vi "DataTypesDetect.vi"(1 "input data":cluster{"name":string, "type desc":i16[]}[](array[cluster])) -> (0 "output data":cluster{"name":string, "type desc":i16[]}[](array[cluster]))   [LabVIEW 2010]
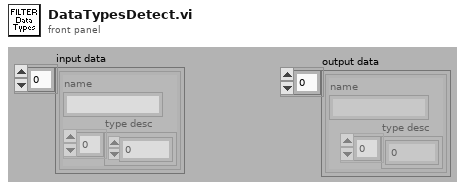
[diagram p1: front panel]
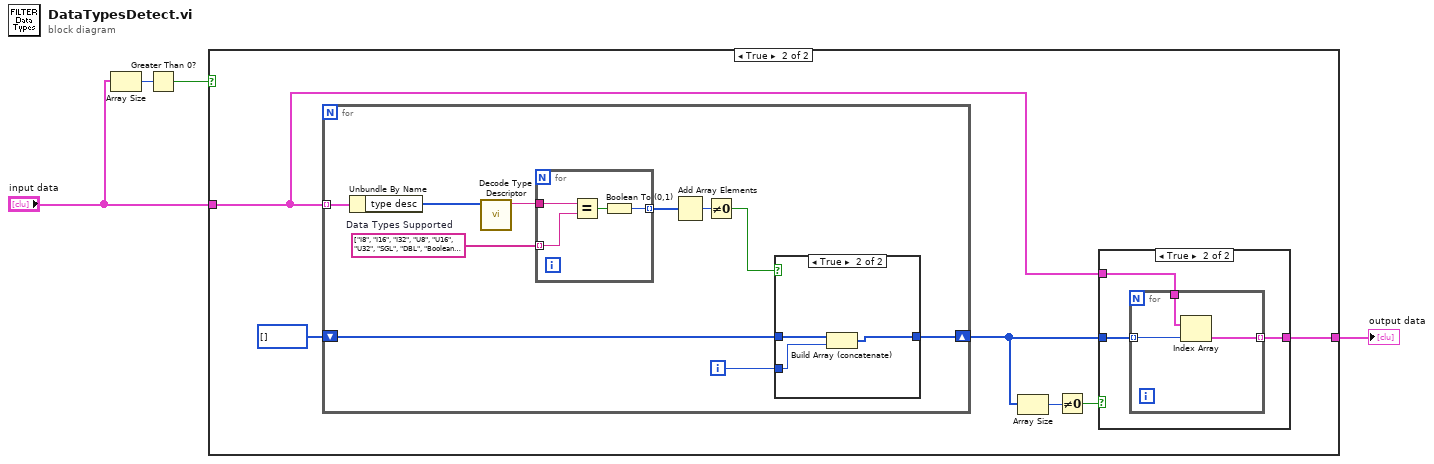
[diagram p0: block diagram]
diagram:
  n1 = Array Size(array="input data") -> (size(s)=w2:i32)
  n2 = Greater Than 0?(x=w2) -> (x > 0?=w3:bool)
  n3 = case shown="True" w3 {
    tunnel: [w5 w11] -> w4
    tunnel: "input data" -> [w5 w8]
    frame False {
    }
    frame True {
      n4 = for {
        tunnel: w8 -> [w27] mode=indexing
        shift-right: [w23] -> w9
        shift-left: i32[] [] -> [w24]
        i -> [w22]
        w21 = string[] ["I8", "I16", "I32", "U8", "U16", "U32", "SGL", "DBL", "Boolean", "String", "Array1D(I8)", "Array1D(I16)", "Array1D(I32)", "Array1D(U8)", "Array1D(U16)", "Array1D(U32)", "Array1D(SGL)", "Array1D(DBL)", "Array1D(Boolean)", "Array1D(String)", "Array2D(I8)", "Array2D(I16)", "Array2D(I32)", "Array2D(U8)", "Array2D(U16)", "Array2D(U32)", "Array2D(SGL)", "Array2D(DBL)", "Array2D(Boolean)", "Array2D(String)"]  # Data Types Supported
        n5 = Unbundle By Name(w27) -> ("type desc"=w20:i16[])
        n6 = call "Decode Type Descriptor.vi"("TypeDesc"=w20) -> ("Type String"=w19:string)  [unwired: 1 in, 5 out]
        n7 = for {
          tunnel: w21 -> [w35] mode=indexing
          tunnel: w19 -> [w36]
          tunnel: [w33] -> w28 mode=indexing
          n8 = Equal?(x=w36, y=w35) -> (x = y?=w34:bool)
          n9 = Boolean To (0,1)(Boolean=w34) -> (0, 1=w33:i16)
        }
        n10 = Add Array Elements(numeric array=w28) -> (sum=w26:i16)
        n11 = Not Equal To 0?(x=w26) -> (x != 0?=w25:bool)
        n12 = case shown="True" w25 {
          tunnel: w24 -> [w29 w32]
          tunnel: [w29 w30] -> w23
          tunnel: w22 -> [_ w31]
          frame False {
          }
          frame True {
            n13 = Build Array (concatenate)(w32, w31) -> (w30:i32[])
          }
        }
      }
      n14 = Array Size(array=w9) -> (size(s)=w6:i32)
      n15 = Not Equal To 0?(x=w6) -> (x != 0?=w7:bool)
      n16 = case shown="True" w7 {
        tunnel: [w12 w13] -> w11
        tunnel: w9 -> [_ w15]
        tunnel: w8 -> [w12 w14]
        frame False {
        }
        frame True {
          n17 = for {
            tunnel: w15 -> [w17] mode=indexing
            tunnel: w14 -> [w18]
            tunnel: [w16] -> w13 mode=indexing
            n18 = Index Array(array=w18, index=w17) -> (element=w16:cluster{"name":string, "type desc":i16[]})
          }
        }
      }
    }
  }
  "output data" <- w4
